vi "Serial_WriteLines.vi"(8 "error in (no error)":errorcluster, 9 "REPL":string, 10 "Send":string, 11 "Python in":cluster{"Python":refnum<k35>, "py file":path}) -> (0 "error out":errorcluster, 1 "Rest":string, 3 "Python out":cluster{"Python":refnum<k35>, "py file":path})   [LabVIEW 2020]
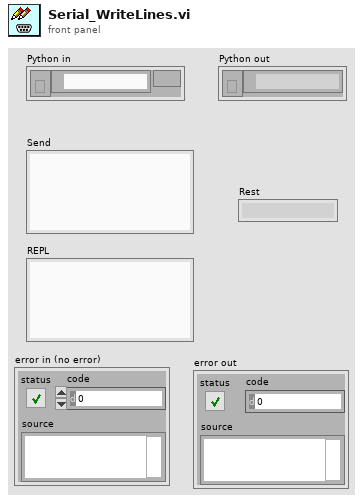
[diagram p1: front panel]
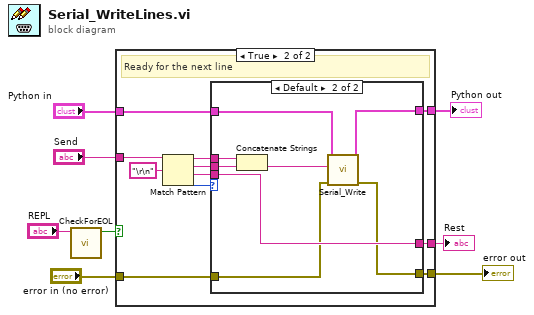
[diagram p0: block diagram]
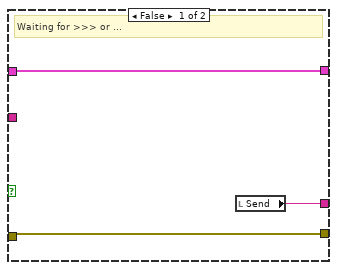
[diagram p2: hidden frame]
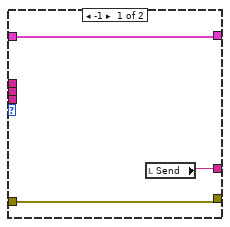
[diagram p3: hidden frame]
diagram:
  n1 = call "CheckForEOL.vi"("REPL"="REPL") -> ("Complete?"=w2:bool)  [unwired: 10 in]
  n2 = case shown="True" w2 {
    tunnel: "Send" -> [_ w21]
    tunnel: [w11 w17] -> w7
    tunnel: "Python in" -> [w9 w15]
    tunnel: "error in (no error)" -> [w10 w14]
    tunnel: [w10 w13] -> w4
    tunnel: [w9 w12] -> w3
    frame False {
      # "Waiting for >>> or ..."
      n3 = local read "Send"() -> (w11:string)
    }
    frame True {
      # "Ready for the next line"
      n4 = Match Pattern(string=w21, regular expression="\r\n") -> (before substring=w22:string, match substring=w20:string, after substring=w16:string, offset past match=w18:i32)  [unwired: 1 in]
      n5 = case shown="Default" w18 {
        tunnel: w22 -> [_ w33]
        tunnel: w20 -> [_ w32]
        tunnel: w15 -> [w23 w27]
        tunnel: [w25 w31] -> w17
        tunnel: w16 -> [_ w31]
        tunnel: w14 -> [w24 w29]
        tunnel: [w24 w28] -> w13
        tunnel: [w23 w26] -> w12
        frame -1 {
          n6 = local read "Send"() -> (w25:string)
        }
        frame Default {
          n7 = Concatenate Strings(w33, w32) -> (w30:string)
          n8 = call "Serial_Write.vi"("error in (no error)"=w29, "Text to write"=w30, "Python in"=w27) -> ("error out"=w28:errorcluster, "Python out"=w26:cluster{"Python":refnum<k35>, "py file":path})  [unwired: 7 in]
        }
      }
    }
  }
  "Python out" <- w3
  "Rest" <- w7
  "error out" <- w4
